vi "PDMS OB AV Module.vi"(1 "Right":bool, 3 "Error In":errorcluster, 4 "Arm":enum32{"meArm", "uArm"}(ring), 5 "Left":bool, 6 "FPGA VI Reference In":refnum<k20>) -> (0 "Error Out":errorcluster, 2 "FPGA VI Reference Out":refnum<k20>)   [LabVIEW 2015]
uses:
  <vilib>/Utility/error.llb/Error Cluster From Error Code.vi
  <vilib>/rvi/errors/niLvFpgaAdjustHostInterfaceError.vi
  Utilities/RT GV.vi
  <vilib>/rvi/interface/nirviReadWriteControl/nirviReadWriteControl.xnode
  NiFpgaLv.dll
  <vilib>/rvi/interface/Simulation/niFpgaSimulationCallBeginRW.vi
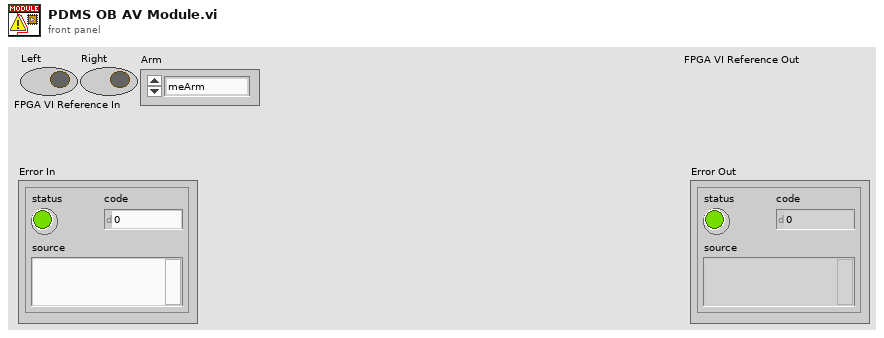
[diagram p1: front panel]
types:
  T1 = cluster{"Motor Speed Left":i16, "Motor Speed Right":i16}
  T2 = enum16{"Stop", "LED", "Front", "Back", "Left", "Right"}
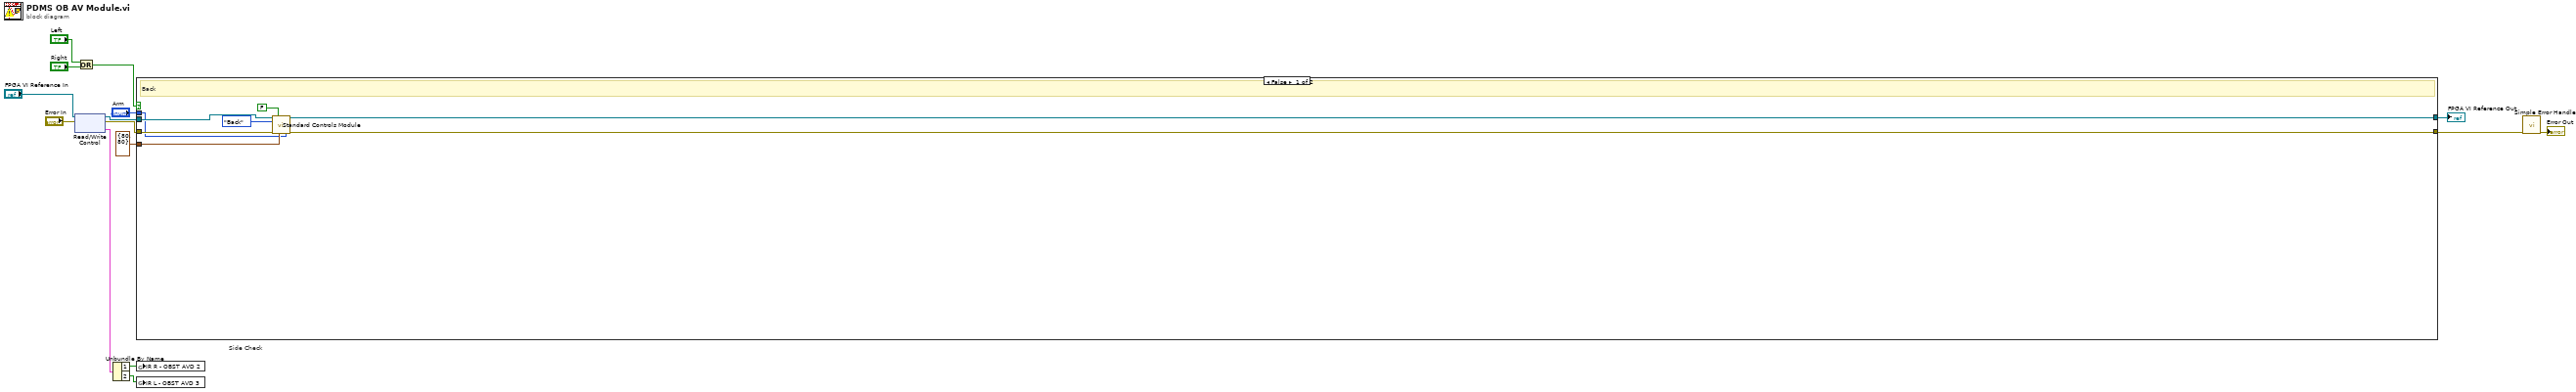
[diagram p0: block diagram]
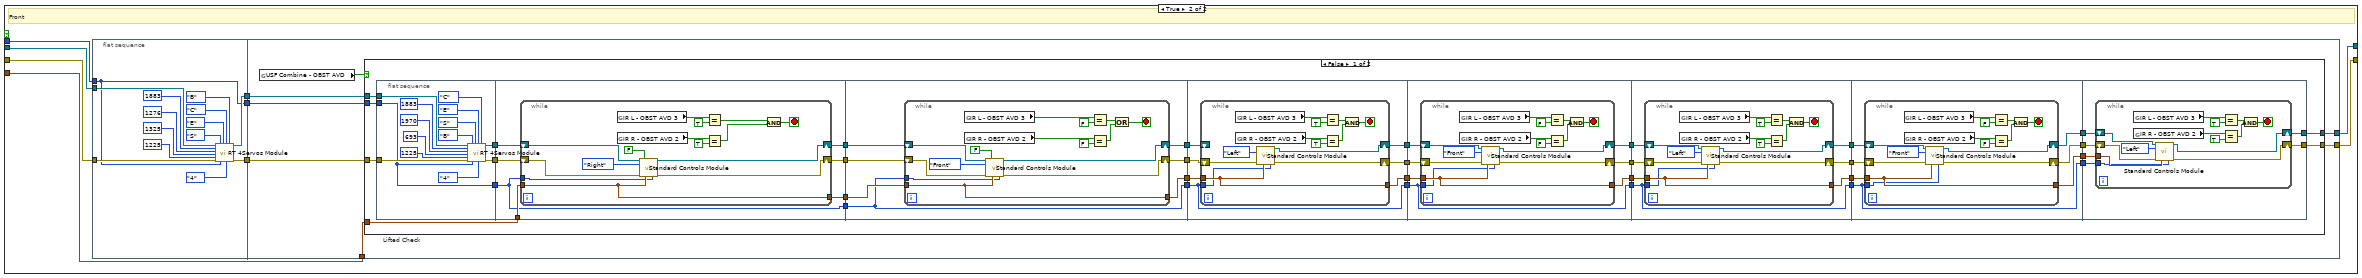
[diagram p2: hidden frame]
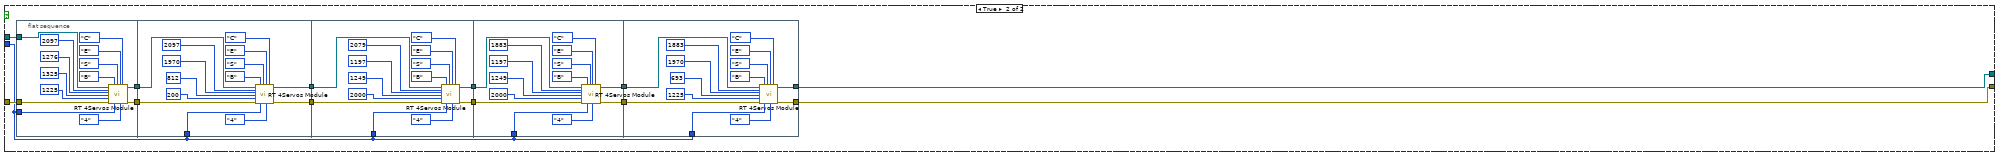
[diagram p3: hidden frame]
diagram:
  # "Side Check"
  n1 = xnode "Read/Write Control"("FPGA VI Reference In"="FPGA VI Reference In", "error in"="Error In") -> ("FPGA VI Reference Out"=w4:refnum<k20>, "error out"=w6:errorcluster, "IR"=w15:cluster{"1":bool, "2":bool})
  n2 = Or(x="Left", y="Right") -> (x .or. y?=w10:bool)
  n3 = Unbundle By Name(w15) -> ("1"=w14:bool, "2"=w13:bool)
  n4 = case shown="False" w10 {
    tunnel: w6 -> [w23 w31]
    tunnel: [w20 w30] -> w7
    tunnel: [w19 w29] -> w5
    tunnel: w4 -> [w18 w28]
    tunnel: T1 {"Motor Speed Left"=80, "Motor Speed Right"=80} ("Speed") -> [w17 w27]
    tunnel: "Arm" -> [w16 w25]
    frame False {
      # "Back"
      n5 = call "Standard Controls Module.vi"("FPGA VI Reference In"=w18, "Control Type"=FALSE, "Command"=T2."Back", "Error In"=w23, "Speed"=w17, "Arm"=w16) -> ("FPGA VI Reference Out"=w19:refnum<k20>, "Error Out"=w20:errorcluster)  [unwired: 7 in, 1 out]
    }
    frame True {
      # "Front"
      n6 = flat-sequence {
        tunnel: w31 -> [w46]
        tunnel: [w36] -> w32
        tunnel: w28 -> [w34]
        tunnel: [w35] -> w26
        tunnel: w25 -> [w33]
        tunnel: [w33] -> w24
        tunnel: w32 -> [w53]
        tunnel: [w51] -> w30
        tunnel: [w50] -> w29
        tunnel: w27 -> [w49]
        tunnel: w26 -> [w48]
        tunnel: w24 -> [w47]
        frame #0 {
          n7 = call "RT 4Servos Module.vi"("FPGA VI Reference In"=w34, "Angle 1"=i64 1883, "Angle 2"=i64 1276, "Angle 3"=i64 1325, "Angle 4"=i64 1225, "Error In"=w46, "Motor 1"=enum16{"B", "S", "E", "C"}."S", "Arm"=w33, "Motor 2"=enum16{"B", "S", "E", "C"}."E", "Motor 3"=enum16{"B", "S", "E", "C"}."C", "No. of Motors"=enum16{"1", "2", "3", "4"}."4", "Motor 4"=enum16{"B", "S", "E", "C"}."B") -> ("FPGA VI Reference Out"=w35:refnum<k20>, "Error Out"=w36:errorcluster)  [unwired: 6 in]
        }
        frame #1 {
          # "Lifted Check"
          n8 = global read "RT GV.vi" "USF Combine - OBST AVD"() -> (w52:bool)
          n9 = case shown="False" w52 {
            tunnel: w53 -> [w86 w260]
            tunnel: [w72 w256] -> w51
            tunnel: [w71 w249] -> w50
            tunnel: w49 -> [w70 _]
            tunnel: w48 -> [w62 w254]
            tunnel: w47 -> [w61 w248]
            frame False {
              n10 = flat-sequence {
                tunnel: w86 -> [w100]
                tunnel: [w90] -> w85
                tunnel: [w89] -> w63
                tunnel: w62 -> [w88]
                tunnel: w61 -> [w87]
                tunnel: [w87] -> w60
                tunnel: w85 -> [w107]
                tunnel: [w105] -> w84
                tunnel: [w106] -> w83
                tunnel: w70 -> [w104]
                tunnel: [w103] -> w69
                tunnel: w63 -> [w102]
                tunnel: w60 -> [w101]
                tunnel: [w101] -> w59
                tunnel: w84 -> [w129]
                tunnel: w83 -> [w128]
                tunnel: [w126] -> w82
                tunnel: [w127] -> w81
                tunnel: w69 -> [w125]
                tunnel: [w124] -> w68
                tunnel: w59 -> [w123]
                tunnel: [w123] -> w58
                tunnel: w82 -> [w151]
                tunnel: w81 -> [w150]
                tunnel: [w149] -> w80
                tunnel: [w148] -> w79
                tunnel: w68 -> [w147]
                tunnel: [w146] -> w67
                tunnel: w58 -> [w145]
                tunnel: [w145] -> w57
                tunnel: w80 -> [w171]
                tunnel: w79 -> [w170]
                tunnel: [w169] -> w78
                tunnel: [w168] -> w77
                tunnel: w67 -> [w167]
                tunnel: [w166] -> w66
                tunnel: w57 -> [w165]
                tunnel: [w165] -> w56
                tunnel: w78 -> [w192]
                tunnel: w77 -> [w191]
                tunnel: [w190] -> w76
                tunnel: [w189] -> w75
                tunnel: w66 -> [w188]
                tunnel: [w187] -> w65
                tunnel: w56 -> [w186]
                tunnel: [w186] -> w55
                tunnel: w76 -> [w213]
                tunnel: w75 -> [w212]
                tunnel: [w211] -> w74
                tunnel: [w210] -> w73
                tunnel: w65 -> [w209]
                tunnel: [w208] -> w64
                tunnel: w55 -> [w207]
                tunnel: [w207] -> w54
                tunnel: w74 -> [w233]
                tunnel: w73 -> [w232]
                tunnel: [w231] -> w72
                tunnel: [w230] -> w71
                tunnel: w64 -> [w229]
                tunnel: w54 -> [w228]
                frame #0 {
                  n11 = call "RT 4Servos Module.vi"("FPGA VI Reference In"=w88, "Angle 1"=i64 1883, "Angle 2"=i64 1970, "Angle 3"=i64 693, "Angle 4"=i64 1225, "Error In"=w100, "Motor 1"=enum16{"B", "S", "E", "C"}."B", "Arm"=w87, "Motor 2"=enum16{"B", "S", "E", "C"}."S", "Motor 3"=enum16{"B", "S", "E", "C"}."E", "No. of Motors"=enum16{"1", "2", "3", "4"}."4", "Motor 4"=enum16{"B", "S", "E", "C"}."C") -> ("FPGA VI Reference Out"=w89:refnum<k20>, "Error Out"=w90:errorcluster)  [unwired: 6 in]
                }
                frame #1 {
                  n12 = while {
                    shift-right: [w110] -> w105
                    shift-left: w102 -> [w111]
                    shift-right: [w112] -> w106
                    shift-left: w107 -> [w122]
                    tunnel: w104 -> [w109]
                    tunnel: [w109] -> w103
                    tunnel: w101 -> [w108]
                    stop <- w115 stop-if-true
                    n13 = global read "RT GV.vi" "IR L - OBST AVD 3"() -> (w114:bool)
                    n14 = global read "RT GV.vi" "IR R - OBST AVD 2"() -> (w113:bool)
                    n15 = call "Standard Controls Module.vi"("FPGA VI Reference In"=w111, "Control Type"=FALSE, "Command"=T2."Right", "Error In"=w122, "Speed"=w109, "Arm"=w108) -> ("FPGA VI Reference Out"=w110:refnum<k20>, "Error Out"=w112:errorcluster)  [unwired: 7 in, 1 out]
                    n16 = Equal?(x=w114, y=TRUE) -> (x = y?=w117:bool)
                    n17 = Equal?(x=w113, y=TRUE) -> (x = y?=w116:bool)
                    n18 = And(x=w117, y=w116) -> (x .and. y?=w115:bool)
                  }
                }
                frame #2 {
                  n19 = while {
                    shift-right: [w133] -> w126
                    shift-left: w129 -> [w132]
                    shift-right: [w134] -> w127
                    shift-left: w128 -> [w144]
                    tunnel: w125 -> [w131]
                    tunnel: [w131] -> w124
                    tunnel: w123 -> [w130]
                    stop <- w137 stop-if-true
                    n20 = global read "RT GV.vi" "IR L - OBST AVD 3"() -> (w142:bool)
                    n21 = global read "RT GV.vi" "IR R - OBST AVD 2"() -> (w143:bool)
                    n22 = call "Standard Controls Module.vi"("FPGA VI Reference In"=w132, "Control Type"=FALSE, "Command"=T2."Front", "Error In"=w144, "Speed"=w131, "Arm"=w130) -> ("FPGA VI Reference Out"=w133:refnum<k20>, "Error Out"=w134:errorcluster)  [unwired: 7 in, 1 out]
                    n23 = Equal?(x=w142, y=FALSE) -> (x = y?=w140:bool)
                    n24 = Equal?(x=w143, y=FALSE) -> (x = y?=w141:bool)
                    n25 = Or(x=w140, y=w141) -> (x .or. y?=w137:bool)
                  }
                }
                frame #3 {
                  n26 = while {
                    shift-right: [w154] -> w149
                    shift-left: w151 -> [_]
                    shift-right: [w155] -> w148
                    shift-left: w150 -> [w157]
                    tunnel: w147 -> [w153]
                    tunnel: [w153] -> w146
                    tunnel: w145 -> [w152]
                    stop <- w158 stop-if-true
                    n27 = global read "RT GV.vi" "IR L - OBST AVD 3"() -> (w160:bool)
                    n28 = global read "RT GV.vi" "IR R - OBST AVD 2"() -> (w159:bool)
                    n29 = call "Standard Controls Module.vi"("Command"=T2."Left", "Error In"=w157, "Speed"=w153, "Arm"=w152) -> ("FPGA VI Reference Out"=w154:refnum<k20>, "Error Out"=w155:errorcluster)  [unwired: 9 in, 1 out]
                    n30 = Equal?(x=w160, y=TRUE) -> (x = y?=w162:bool)
                    n31 = Equal?(x=w159, y=TRUE) -> (x = y?=w161:bool)
                    n32 = And(x=w162, y=w161) -> (x .and. y?=w158:bool)
                  }
                }
                frame #4 {
                  n33 = while {
                    shift-right: [w174] -> w169
                    shift-left: w171 -> [w175]
                    shift-right: [w176] -> w168
                    shift-left: w170 -> [w178]
                    tunnel: w167 -> [w173]
                    tunnel: [w173] -> w166
                    tunnel: w165 -> [w172]
                    stop <- w179 stop-if-true
                    n34 = global read "RT GV.vi" "IR L - OBST AVD 3"() -> (w181:bool)
                    n35 = global read "RT GV.vi" "IR R - OBST AVD 2"() -> (w180:bool)
                    n36 = call "Standard Controls Module.vi"("FPGA VI Reference In"=w175, "Command"=T2."Front", "Error In"=w178, "Speed"=w173, "Arm"=w172) -> ("FPGA VI Reference Out"=w174:refnum<k20>, "Error Out"=w176:errorcluster)  [unwired: 8 in, 1 out]
                    n37 = Equal?(x=w181, y=FALSE) -> (x = y?=w183:bool)
                    n38 = Equal?(x=w180, y=FALSE) -> (x = y?=w182:bool)
                    n39 = And(x=w183, y=w182) -> (x .and. y?=w179:bool)
                  }
                }
                frame #5 {
                  n40 = while {
                    shift-right: [w196] -> w190
                    shift-left: w192 -> [w195]
                    shift-right: [w197] -> w189
                    shift-left: w191 -> [w199]
                    tunnel: w188 -> [w194]
                    tunnel: [w194] -> w187
                    tunnel: w186 -> [w193]
                    stop <- w200 stop-if-true
                    n41 = global read "RT GV.vi" "IR L - OBST AVD 3"() -> (w202:bool)
                    n42 = global read "RT GV.vi" "IR R - OBST AVD 2"() -> (w201:bool)
                    n43 = call "Standard Controls Module.vi"("FPGA VI Reference In"=w195, "Command"=T2."Left", "Error In"=w199, "Speed"=w194, "Arm"=w193) -> ("FPGA VI Reference Out"=w196:refnum<k20>, "Error Out"=w197:errorcluster)  [unwired: 8 in, 1 out]
                    n44 = Equal?(x=w202, y=TRUE) -> (x = y?=w204:bool)
                    n45 = Equal?(x=w201, y=TRUE) -> (x = y?=w203:bool)
                    n46 = And(x=w204, y=w203) -> (x .and. y?=w200:bool)
                  }
                }
                frame #6 {
                  n47 = while {
                    shift-right: [w216] -> w211
                    shift-left: w213 -> [w217]
                    shift-right: [w218] -> w210
                    shift-left: w212 -> [w220]
                    tunnel: w209 -> [w215]
                    tunnel: [w215] -> w208
                    tunnel: w207 -> [w214]
                    stop <- w221 stop-if-true
                    n48 = global read "RT GV.vi" "IR L - OBST AVD 3"() -> (w223:bool)
                    n49 = global read "RT GV.vi" "IR R - OBST AVD 2"() -> (w222:bool)
                    n50 = call "Standard Controls Module.vi"("FPGA VI Reference In"=w217, "Command"=T2."Front", "Error In"=w220, "Speed"=w215, "Arm"=w214) -> ("FPGA VI Reference Out"=w216:refnum<k20>, "Error Out"=w218:errorcluster)  [unwired: 8 in, 1 out]
                    n51 = Equal?(x=w223, y=FALSE) -> (x = y?=w225:bool)
                    n52 = Equal?(x=w222, y=FALSE) -> (x = y?=w224:bool)
                    n53 = And(x=w225, y=w224) -> (x .and. y?=w221:bool)
                  }
                }
                frame #7 {
                  n54 = while {
                    shift-right: [w237] -> w230
                    shift-left: w233 -> [w236]
                    shift-right: [w238] -> w231
                    shift-left: w232 -> [w240]
                    tunnel: w229 -> [w235]
                    tunnel: w228 -> [w234]
                    stop <- w241 stop-if-true
                    n55 = global read "RT GV.vi" "IR L - OBST AVD 3"() -> (w243:bool)
                    n56 = global read "RT GV.vi" "IR R - OBST AVD 2"() -> (w242:bool)
                    n57 = call "Standard Controls Module.vi"("FPGA VI Reference In"=w236, "Command"=T2."Left", "Error In"=w240, "Speed"=w235, "Arm"=w234) -> ("FPGA VI Reference Out"=w237:refnum<k20>, "Error Out"=w238:errorcluster)  [unwired: 8 in, 1 out]
                    n58 = Equal?(x=w243, y=TRUE) -> (x = y?=w245:bool)
                    n59 = Equal?(x=w242, y=TRUE) -> (x = y?=w244:bool)
                    n60 = And(x=w245, y=w244) -> (x .and. y?=w241:bool)
                  }
                }
              }
            }
            frame True {
              n61 = flat-sequence {
                tunnel: w260 -> [w265]
                tunnel: [w264] -> w257
                tunnel: w254 -> [w263]
                tunnel: [w262] -> w253
                tunnel: w248 -> [w261]
                tunnel: [w279] -> w258
                tunnel: w257 -> [w278]
                tunnel: w253 -> [w277]
                tunnel: [w276] -> w252
                tunnel: w248 -> [w275]
                tunnel: [w293] -> w259
                tunnel: w258 -> [w292]
                tunnel: w252 -> [w291]
                tunnel: [w290] -> w251
                tunnel: w248 -> [w289]
                tunnel: w259 -> [w307]
                tunnel: [w306] -> w255
                tunnel: w251 -> [w305]
                tunnel: [w304] -> w250
                tunnel: w248 -> [w303]
                tunnel: [w330] -> w256
                tunnel: w255 -> [w329]
                tunnel: w250 -> [w319]
                tunnel: [w318] -> w249
                tunnel: w248 -> [w317]
                frame #0 {
                  n62 = call "RT 4Servos Module.vi"("FPGA VI Reference In"=w263, "Angle 1"=i64 2097, "Angle 2"=i64 1276, "Angle 3"=i64 1325, "Angle 4"=i64 1225, "Error In"=w265, "Motor 1"=enum16{"B", "S", "E", "C"}."B", "Arm"=w261, "Motor 2"=enum16{"B", "S", "E", "C"}."S", "Motor 3"=enum16{"B", "S", "E", "C"}."E", "No. of Motors"=enum16{"1", "2", "3", "4"}."4", "Motor 4"=enum16{"B", "S", "E", "C"}."C") -> ("FPGA VI Reference Out"=w262:refnum<k20>, "Error Out"=w264:errorcluster)  [unwired: 6 in]
                }
                frame #1 {
                  n63 = call "RT 4Servos Module.vi"("FPGA VI Reference In"=w277, "Angle 1"=i64 2097, "Angle 2"=i64 1970, "Angle 3"=i64 812, "Angle 4"=i64 200, "Error In"=w278, "Motor 1"=enum16{"B", "S", "E", "C"}."B", "Arm"=w275, "Motor 2"=enum16{"B", "S", "E", "C"}."S", "Motor 3"=enum16{"B", "S", "E", "C"}."E", "No. of Motors"=enum16{"1", "2", "3", "4"}."4", "Motor 4"=enum16{"B", "S", "E", "C"}."C") -> ("FPGA VI Reference Out"=w276:refnum<k20>, "Error Out"=w279:errorcluster)  [unwired: 6 in]
                }
                frame #2 {
                  n64 = call "RT 4Servos Module.vi"("FPGA VI Reference In"=w291, "Angle 1"=i64 2079, "Angle 2"=i64 1197, "Angle 3"=i64 1249, "Angle 4"=i64 2000, "Error In"=w292, "Motor 1"=enum16{"B", "S", "E", "C"}."B", "Arm"=w289, "Motor 2"=enum16{"B", "S", "E", "C"}."S", "Motor 3"=enum16{"B", "S", "E", "C"}."E", "No. of Motors"=enum16{"1", "2", "3", "4"}."4", "Motor 4"=enum16{"B", "S", "E", "C"}."C") -> ("FPGA VI Reference Out"=w290:refnum<k20>, "Error Out"=w293:errorcluster)  [unwired: 6 in]
                }
                frame #3 {
                  n65 = call "RT 4Servos Module.vi"("FPGA VI Reference In"=w305, "Angle 1"=i64 1883, "Angle 2"=i64 1197, "Angle 3"=i64 1249, "Angle 4"=i64 2000, "Error In"=w307, "Motor 1"=enum16{"B", "S", "E", "C"}."B", "Arm"=w303, "Motor 2"=enum16{"B", "S", "E", "C"}."S", "Motor 3"=enum16{"B", "S", "E", "C"}."E", "No. of Motors"=enum16{"1", "2", "3", "4"}."4", "Motor 4"=enum16{"B", "S", "E", "C"}."C") -> ("FPGA VI Reference Out"=w304:refnum<k20>, "Error Out"=w306:errorcluster)  [unwired: 6 in]
                }
                frame #4 {
                  n66 = call "RT 4Servos Module.vi"("FPGA VI Reference In"=w319, "Angle 1"=i64 1883, "Angle 2"=i64 1970, "Angle 3"=i64 693, "Angle 4"=i64 1225, "Error In"=w329, "Motor 1"=enum16{"B", "S", "E", "C"}."B", "Arm"=w317, "Motor 2"=enum16{"B", "S", "E", "C"}."S", "Motor 3"=enum16{"B", "S", "E", "C"}."E", "No. of Motors"=enum16{"1", "2", "3", "4"}."4", "Motor 4"=enum16{"B", "S", "E", "C"}."C") -> ("FPGA VI Reference Out"=w318:refnum<k20>, "Error Out"=w330:errorcluster)  [unwired: 6 in]
                }
              }
            }
          }
        }
      }
    }
  }
  "FPGA VI Reference Out" <- w5
  n67 = global write "RT GV.vi" "IR R - OBST AVD 2"(w14) -> ()
  n68 = global write "RT GV.vi" "IR L - OBST AVD 3"(w13) -> ()
  n69 = call <vilib>:"Simple Error Handler.vi"("error in (no error)"=w7) -> ("error out"=→"Error Out":errorcluster)  [unwired: 4 in, 4 out]
